vi "Tabor 5064 - Trigger (SubVI).vi"(7 "GPIB Address":string="4", 8 "error_in":errorcluster) -> (0 "error_out":errorcluster)   [LabVIEW 2018]
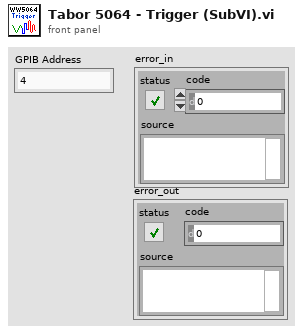
[diagram p1: front panel]
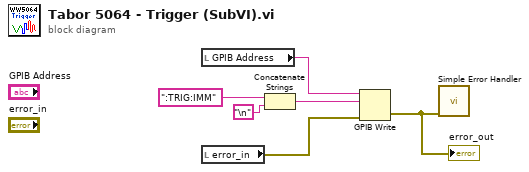
[diagram p0: block diagram]
diagram:
  n1 = local read "GPIB Address"() -> (w4:string)
  n2 = local read "error_in"() -> (w1:errorcluster)
  n3 = Concatenate Strings(":TRIG:IMM" ("format string"), "\n") -> (w2:string)
  n4 = GPIB Write(0:w4, 1:w2, 3:w1) -> (6:w6:errorcluster)  [unwired: 2 in, 1 out]
  "error_out" <- w6
  n5 = call <vilib>:"Simple Error Handler.vi"("error in (no error)"=w6) -> ()  [unwired: 4 in, 5 out]
